vi "ArrayFile.vi"() -> (13 "Array Names":string[](array[string]), 19 "error out":errorcluster)   [LabVIEW 2026]
doc: "This VI checks the names of all arrays in a data file or deletes a given array from a data file."
panel:
  in  "error in":errorcluster
  in  "ArrayName":string
  in  "Path":path
  in  "Read (F)/Delete":bool
  # "This vi checks the names of all arrays in a data file or deletes a given array from a data file. \nSee control descriptions in the diagram for more information."
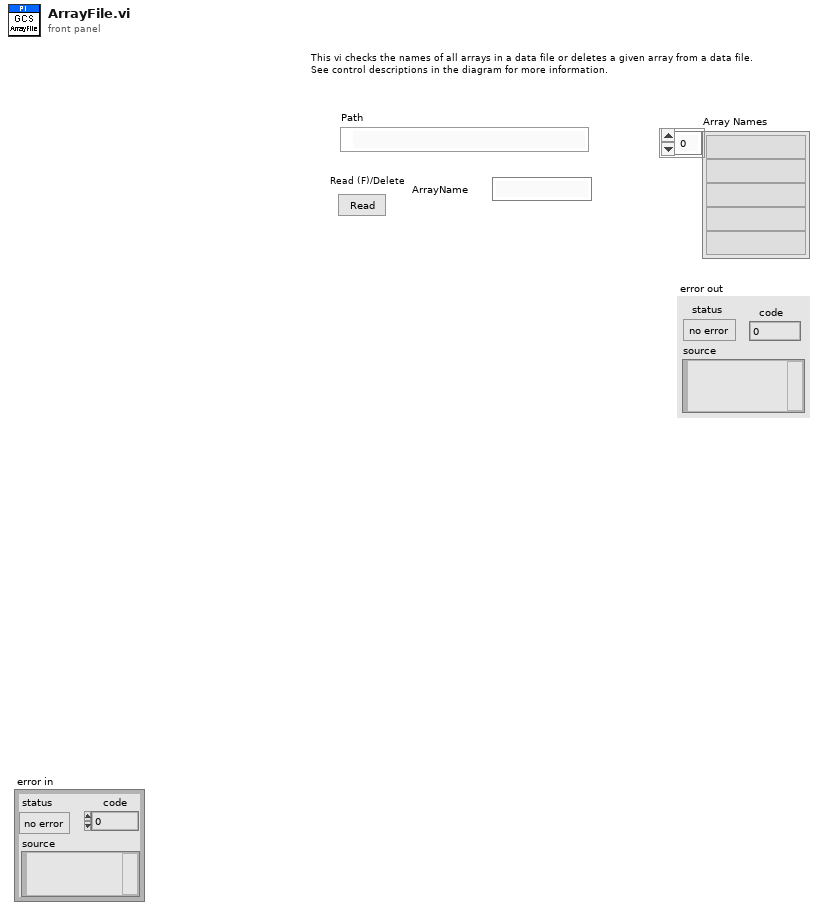
[diagram p1: front panel]
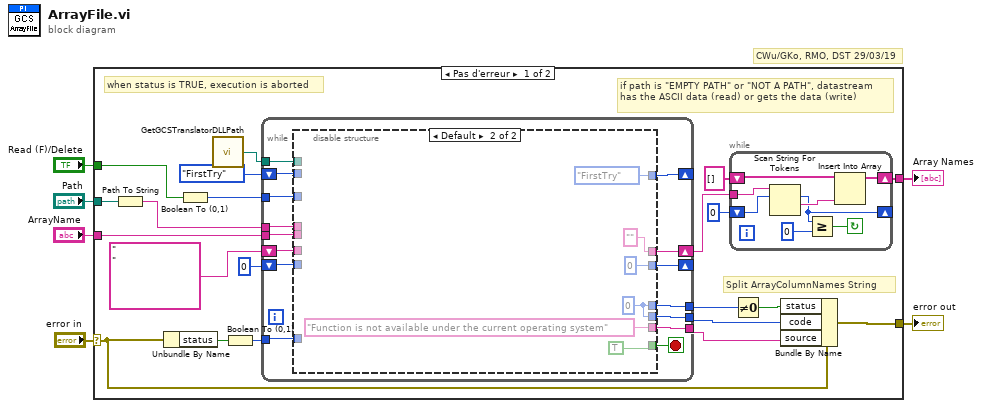
[diagram p0: block diagram]
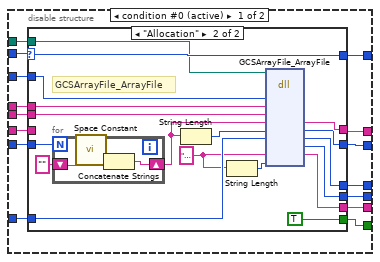
[diagram p2: hidden frame]
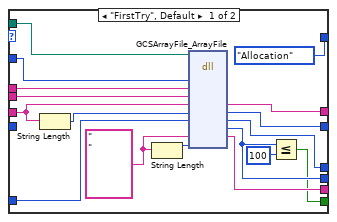
[diagram p3: hidden frame]
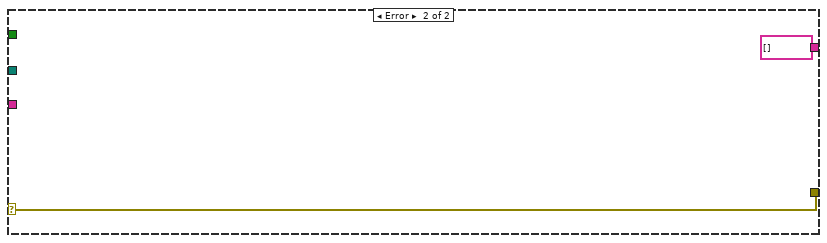
[diagram p4: hidden frame]
diagram:
  # "CWu/GKo, RMO, DST 29/03/19"
  n1 = case shown="Pas d'erreur" "error in" {
    selector: "error in" -> [w11 w110]
    tunnel: [w23 string[] []] -> w6
    tunnel: [w22 w110] -> w5
    tunnel: "Read (F)/Delete" -> [w18 _]
    tunnel: "ArrayName" -> [w13 _]
    tunnel: "Path" -> [w8 _]
    frame No Error {
      # "Split ArrayColumnNames String"
      # "when status is TRUE, execution is aborted"
      # "if path is \"EMPTY PATH\" or \"NOT A PATH\", datastream has the ASCII data (read) or gets the data (write)"
      n2 = Path To String(path=w8) -> (string=w9:string)
      n3 = Unbundle By Name(w11) -> ("status"=w10:bool)
      n4 = Boolean To (0,1)(Boolean=w18) -> (0, 1=w19:i16)
      n5 = call "GetGCSTranslatorDLLPath.vi"() -> ("DLL path"=w7:path)  [unwired: 1 in]
      n6 = Boolean To (0,1)(Boolean=w10) -> (0, 1=w20:i16)
      n7 = while {
        tunnel: w9 -> [w41]
        tunnel: [w40] -> w21
        tunnel: w20 -> [w39]
        tunnel: w19 -> [w38]
        tunnel: [w37] -> w17
        tunnel: [w36] -> w16
        shift-right: [w29] -> _
        shift-left: enum16{"FirstTry", "Allocation"}."FirstTry" -> [w35]
        shift-right: [w42] -> w26
        shift-left: "                                                                                              " ("Array Column Names") -> [w34]
        tunnel: w13 -> [w33]
        shift-right: [w32] -> _
        shift-left: u32 0 ("ColumnameBufferSize") -> [w31]
        tunnel: w7 -> [w28]
        stop <- w30 stop-if-true
        n8 = disable-structure shown="Default" {
          disable-tunnel: [w57 "" ("Array Column Names")] -> w42
          disable-tunnel: w41 -> [w56 _]
          disable-tunnel: [w55 w100] -> w40
          disable-tunnel: w39 -> [w54 _]
          disable-tunnel: w38 -> [w53 _]
          disable-tunnel: [w52 w100] -> w37
          disable-tunnel: [w51 "Function is not available under the current operating system" ("errorsource")] -> w36
          disable-tunnel: w35 -> [w50 _]
          disable-tunnel: w34 -> [w49 _]
          disable-tunnel: w33 -> [w48 _]
          disable-tunnel: [w47 u32 0 ("ColumnameBufferSize")] -> w32
          disable-tunnel: w31 -> [w46 _]
          disable-tunnel: [w45 TRUE] -> w30
          disable-tunnel: [w44 enum16{"FirstTry", "Allocation"}."FirstTry"] -> w29
          disable-tunnel: w28 -> [w43 _]
          frame condition #0 (active) {
            n9 = case shown="\"Allocation\"" w50 {
              selector: w50 -> [_ w77]
              tunnel: [w69 w92] -> w57
              tunnel: w56 -> [w71 w89]
              tunnel: [w59 w88] -> w55
              tunnel: w54 -> [w70 w86]
              tunnel: w53 -> [w60 w85]
              tunnel: [w64 w82] -> w52
              tunnel: [w65 w81] -> w51
              tunnel: w49 -> [w68 _]
              tunnel: w48 -> [w67 w79]
              tunnel: [w66 w76] -> w47
              tunnel: w46 -> [_ w80]
              tunnel: [w62 TRUE] -> w45
              tunnel: [enum16{"FirstTry", "Allocation"}."Allocation" w77] -> w44
              tunnel: w43 -> [w58 w75]
              frame "FirstTry", Default {
                w73 = "                                                                                                                                                                          " ("errorsource")
                n10 = String Length(string=w68) -> (length=w74:i32)
                n11 = String Length(string=w73) -> (length=w72:i32)
                n12 = dll-call lib="T:/Entwicklung/HostSoftware/LabVIEW/GCSDrivers/source/GCS2LabVIEW/Low Level/GCSTranslator.dll" fn="GCSArrayFile_ArrayFile"(path in=w58, "Delete"=w60, "Path"=w71, "ArrayName"=w67, "Array Column Names"=w68, "ColumnameBufferSize"=w74, "error status"=w70, "errorsource"=w73, "errorsrcbufferlen"=w72) -> ("Array Column Names"=w69:string, "ColumnameBufferSize"=w66:u32, "error status"=w59:u8, "errorcode"=w64:i32, "errorsource"=w65:string)  [unwired: 4 in, 6 out]
                n13 = Less Or Equal?(x=w64, y=100) -> (x <= y?=w62:bool)
              }
              frame "Allocation" {
                w84 = "                                                                                                                                                                          " ("errorsource")
                # "GCSArrayFile_ArrayFile"
                n14 = for {
                  N: w80 -> [_]
                  shift-right: [w94] -> w91
                  shift-left: "" -> [w93]
                  n15 = call <vilib>:"Space Constant.vi"() -> ("String"=w95:string)
                  n16 = Concatenate Strings(w95, w93) -> (w94:string)
                }
                n17 = String Length(string=w91) -> (length=w90:i32)
                n18 = String Length(string=w84) -> (length=w83:i32)
                n19 = dll-call lib="T:/Entwicklung/HostSoftware/LabVIEW/GCSDrivers/source/GCS2LabVIEW/Low Level/GCSTranslator.dll" fn="GCSArrayFile_ArrayFile"(path in=w75, "Delete"=w85, "Path"=w89, "ArrayName"=w79, "Array Column Names"=w91, "ColumnameBufferSize"=w90, "error status"=w86, "errorsource"=w84, "errorsrcbufferlen"=w83) -> ("Array Column Names"=w92:string, "ColumnameBufferSize"=w76:u32, "error status"=w88:u8, "errorcode"=w82:i32, "errorsource"=w81:string)  [unwired: 4 in, 6 out]
              }
            }
          }
          frame condition #1 {
            w100 = u8 0 ("error status")
          }
        }
      }
      n20 = while {
        shift-right: [w107] -> w23
        shift-left: string[] [] -> [w106]
        tunnel: w26 -> [w105]
        shift-right: [w102] -> _
        shift-left: 0 ("offset past token") -> [w103]
        stop <- w108 continue-if-true
        n21 = Scan String For Tokens(8:w103, 9:w105) -> (1:w104:string, 2:w102:i32)  [unwired: 6 out]
        n22 = Greater Or Equal?(x=w102, y=0) -> (x >= y?=w108:bool)
        n23 = Insert Into Array(array=w106, new element=w104) -> (w107:string[])  [unwired: 1 in]
      }
      n24 = Not Equal To 0?(x=w21) -> (x != 0?=w27:bool)
      n25 = Bundle By Name(cluster=w11, "status"=w27, "code"=w17, "source"=w16) -> (w22:errorcluster)
    }
    frame Error {
    }
  }
  "error out" <- w5
  "Array Names" <- w6
